vi "sample1(BasicRW XL).vi"() -> ()   [LabVIEW 2011]
panel:
  in  "OffsetTime":u32=20
  out "err":errorcluster caption="エラー出力" {"code" format="%04x"}
  in  "ID":u8=1 max=253
  in  "Baudrate":u32=1000000
  in  "COM":refnum<visa-resource-name> caption="COMポート"
  in  "STOP":bool
  in  "POSITION":u16(knob)
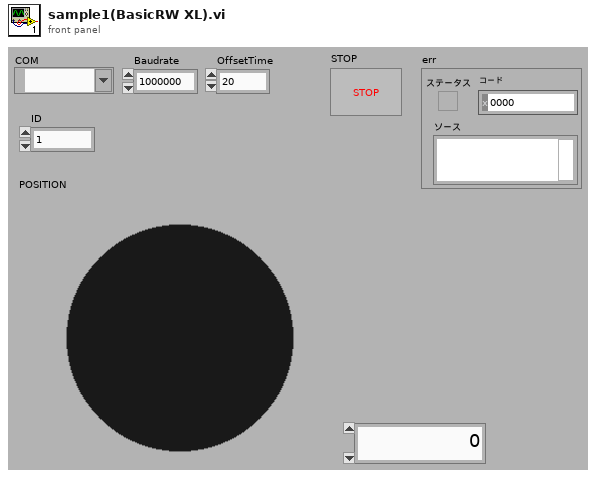
[diagram p1: front panel]
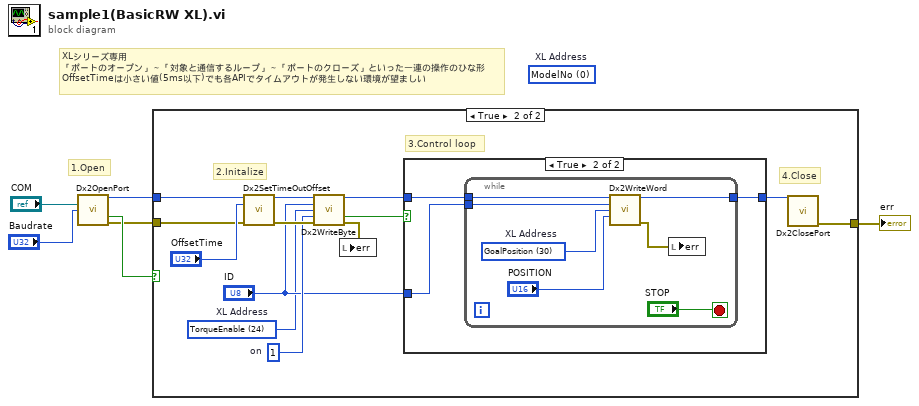
[diagram p0: block diagram]
diagram:
  (unwired) u16 0 items=["ModelNo"=0, "VersionOfFirmware"=2, "ID"=3, "Baudrate"=4, "ReturnDelayTime"=5, "CWAngleLimit"=6, "CCWAngleLimit"=8, "ControlMode"=11, "LimitTemperature"=12, "LowestLimitVoltage"=13, "HighestLimitVoltage"=14, "MaxTorque"=15, "StatusReturnLevel"=17, "AlarmShutdown"=18, "TorqueEnable"=24, "LED"=25, "DGain"=26, "IGain"=27, "PGain"=28, "GoalPosition"=30, "GoalVelocity"=32, "GoalTorque"=35, "PresentPosition"=37, "PresentSPeed"=39, "PresentLoad"=41, "PresentVoltage"=45, "PresentTemperature"=46, "RegistedInstruction"=47, "Moving"=49, "HardwareErrorStatus"=50, "Punch"=51]  # XL Address
  # "1.Open"
  # "XLシリーズ専用\n「ポートのオープン」～「対象と通信するループ」～「ポートのクローズ」といった一連の操作のひな形\nOffsetTimeは小さい値(5ms以下)でも各APIでタイムアウトが発生しない環境が望ましい"
  n1 = call "Dx2OpenPort.vi"("port"="COM", "baudrate"="Baudrate") -> ("dvid"=w3:u32, "成功"=w4:bool, "エラー出力"=w2:errorcluster)  [unwired: 11 in]
  n2 = case shown="TRUE" w4 {
    tunnel: w3 -> [_ w20]
    tunnel: w2 -> [w7 w18]
    tunnel: [w7 w9] -> w1
    frame False {
      # "Fail to open"
    }
    frame True {
      w10 = u16 24 items=["ModelNo"=0, "VersionOfFirmware"=2, "ID"=3, "Baudrate"=4, "ReturnDelayTime"=5, "CWAngleLimit"=6, "CCWAngleLimit"=8, "ControlMode"=11, "LimitTemperature"=12, "LowestLimitVoltage"=13, "HighestLimitVoltage"=14, "MaxTorque"=15, "StatusReturnLevel"=17, "AlarmShutdown"=18, "TorqueEnable"=24, "LED"=25, "DGain"=26, "IGain"=27, "PGain"=28, "GoalPosition"=30, "GoalVelocity"=32, "GoalTorque"=35, "PresentPosition"=37, "PresentSPeed"=39, "PresentLoad"=41, "PresentVoltage"=45, "PresentTemperature"=46, "RegistedInstruction"=47, "Moving"=49, "HardwareErrorStatus"=50, "Punch"=51]  # XL Address
      w13 = u8 1  # on
      # "4.Close"
      # "3.Control loop"
      # "2.Initalize"
      n3 = call "Dx2SetTimeOutOffset.vi"("dvid in"=w20, "OffsetTime"="OffsetTime", "エラー入力"=w18) -> ("dvid out"=w17:u32, "エラー出力"=w15:errorcluster)  [unwired: 11 in]
      n4 = call "Dx2WriteByte.vi"("dvid in"=w17, "id"="ID", "address"=w10, "data in"=w13, "エラー入力"=w15) -> ("dvid out"=w14:u32, "成功"=w16:bool, "エラー出力"=w8:errorcluster)  [unwired: 8 in]
      n5 = local write "err"(w8) -> ()
      n6 = case shown="TRUE" w16 {
        tunnel: w14 -> [w21 w24]
        tunnel: "ID" -> [_ w23]
        tunnel: [w21 w22] -> w11
        frame False {
          # "Fail to initalize"
        }
        frame True {
          n7 = while {
            tunnel: w24 -> [w31]
            tunnel: w23 -> [w30]
            tunnel: [w28] -> w22
            stop <- "STOP" stop-if-true
            w26 = u16 30 items=["ModelNo"=0, "VersionOfFirmware"=2, "ID"=3, "Baudrate"=4, "ReturnDelayTime"=5, "CWAngleLimit"=6, "CCWAngleLimit"=8, "ControlMode"=11, "LimitTemperature"=12, "LowestLimitVoltage"=13, "HighestLimitVoltage"=14, "MaxTorque"=15, "StatusReturnLevel"=17, "AlarmShutdown"=18, "TorqueEnable"=24, "LED"=25, "DGain"=26, "IGain"=27, "PGain"=28, "GoalPosition"=30, "GoalVelocity"=32, "GoalTorque"=35, "PresentPosition"=37, "PresentSPeed"=39, "PresentLoad"=41, "PresentVoltage"=45, "PresentTemperature"=46, "RegistedInstruction"=47, "Moving"=49, "HardwareErrorStatus"=50, "Punch"=51]  # XL Address
            n8 = call "Dx2WriteWord.vi"("dvid in"=w31, "id"=w30, "address"=w26, "data in"="POSITION") -> ("dvid out"=w28:u32, "エラー出力"=w25:errorcluster)  [unwired: 9 in, 1 out]
            n9 = local write "err"(w25) -> ()
          }
        }
      }
      n10 = call "Dx2ClosePort.vi"("dvid"=w11) -> ("エラー出力"=w9:errorcluster)  [unwired: 13 in, 1 out]
    }
  }
  "err" <- w1
